vi "1.vi"(11 "文字列入力":string) -> (3 "文字列出力":string)   [LabVIEW 2019]
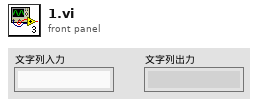
[diagram p1: front panel]
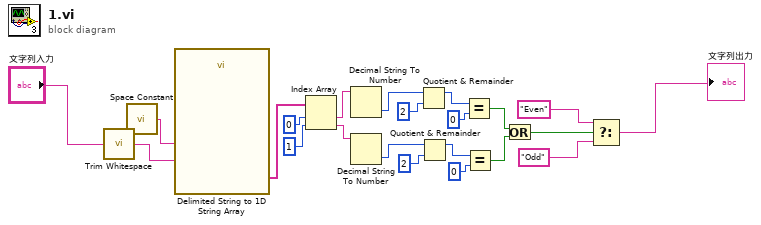
[diagram p0: block diagram]
diagram:
  n1 = call <vilib>:"Trim Whitespace.vi"("string"="文字列入力") -> ("trimmed string"=w6:string)  [unwired: 1 in]
  n2 = call <vilib>:"Space Constant.vi"() -> ("String"=w5:string)
  n3 = call <vilib>:"Delimited String to 1D String Array.vi"("delimiter"=w5, "delimited string"=w6) -> ("string array"=w11:string[])  [unwired: 9 in]
  n4 = Index Array(array=w11, index #1=0, index #2=1) -> (element #1=w8:string, element #2=w7:string)
  n5 = Decimal String To Number(string=w8) -> (number=w12:i32)  [unwired: 2 in, 1 out]
  n6 = Decimal String To Number(string=w7) -> (number=w18:i32)  [unwired: 2 in, 1 out]
  n7 = Quotient & Remainder(x=w12, y=2) -> (x-y*floor(x/y)=w15:i32)  [unwired: 1 out]
  n8 = Quotient & Remainder(x=w18, y=2) -> (x-y*floor(x/y)=w19:i32)  [unwired: 1 out]
  n9 = Equal?(x=w15, y=0) -> (x = y?=w20:bool)
  n10 = Equal?(x=w19, y=0) -> (x = y?=w21:bool)
  n11 = Or(x=w20, y=w21) -> (x .or. y?=w4:bool)
  n12 = Select(t="Even", s=w4, f="Odd") -> (s? t:f=→"文字列出力":string)
